vi "Stop Core.vi"(10 "final error code":i32, 11 "Fluke 2625A (Hydra II) in":refnum<class "Fluke 2625A (Hydra II).lvclass">) -> (3 "Fluke 2625A (Hydra II) out":refnum<class "Fluke 2625A (Hydra II).lvclass">)   [LabVIEW 2013, in "Generic Data Logger.lvlib" / "Fluke 2625A (Hydra II).lvlib" / "Fluke 2625A (Hydra II).lvclass"]
doc: "(<B>Filename</B>: Actor Framework.lvlib:Actor.lvclass:Stop Core.vi)\n\nDefines what the actor does before it stops. Use the <B>final error code</B> input to determine whether the actor shut down in response to an error.\n\nBy default, this method does nothing. A descendant class may override it to define behavior, such as shutting down any processes the actor initiated in its override of the Actor Core method."
uses:
  Fluke 2625A (Hydra II).lvclass
  Generic Data Logger Class/Generic Data Logger.lvclass
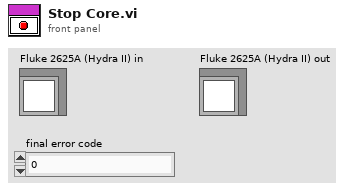
[diagram p1: front panel]
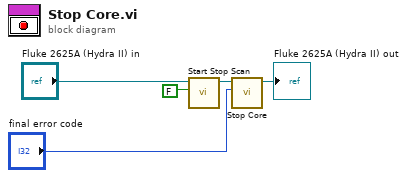
[diagram p0: block diagram]
diagram:
  n1 = call "Start Stop Scan.vi"("Start/Stop"=FALSE, "Generic Data Logger.lvlib:Fluke 2625A (Hydra II).lvlib:Fluke 2625A (Hydra II).lvclass"="Fluke 2625A (Hydra II) in") -> ("Generic Instrument out"=w2:refnum<class "Fluke 2625A (Hydra II).lvclass">)  [unwired: 8 in, 1 out]
  n2 = call-parent "Stop Core.vi"("final error code"="final error code", "Actor in"=w2) -> ("Actor out"=→"Fluke 2625A (Hydra II) out":refnum<class "Fluke 2625A (Hydra II).lvclass">)  [unwired: 9 in]
